vi "Create channel.vi"(8 "error in (no error)":errorcluster, 10 "Lines":T1[](array[typedef])=[1] items=["DIO1...8"=1, "DIO9...16"=2, "DIO17...24"=3, "DIO25...32"=4], 11 "Connection ID":i32=-1) -> (0 "error out":errorcluster, 3 "MicroDAQ.lvlib:Digital output.lvclass":refnum<class "Digital output.lvclass">)   [LabVIEW 2009, in "MicroDAQ.lvlib" / "Digital output.lvclass"]
uses:
  <instrlib>/MicroDAQ/Channel/Digital output/Digital output.lvclass
  <instrlib>/MicroDAQ/Tools/Digital IO channels.ctl
  <instrlib>/MicroDAQ/Channel/Channel.lvclass
  <instrlib>/MicroDAQ/Tools/DIO set direction argument.ctl
  <instrlib>/MicroDAQ/MicroDAQ.lvlib
  <instrlib>/MicroDAQ/Mlink library wraper/mlink.lvlib
  <instrlib>/MicroDAQ/Channel/Digital Input/Digital Input.lvclass
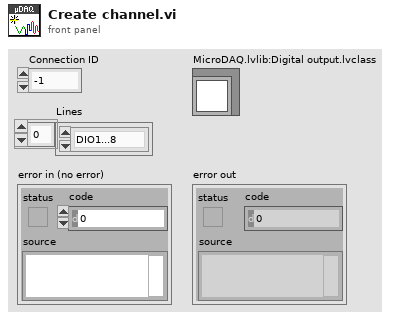
[diagram p1: front panel]
types:
  T1 = typedef "MicroDAQ.lvlib/Digital IO channels.ctl" = u8
  T2 = typedef "MicroDAQ.lvlib/DIO set direction argument.ctl" = enum8{"Input", "Output"}
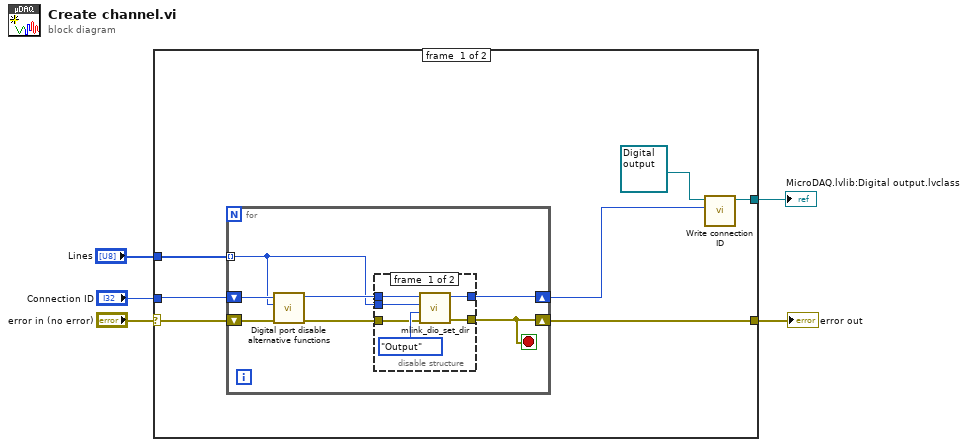
[diagram p0: block diagram]
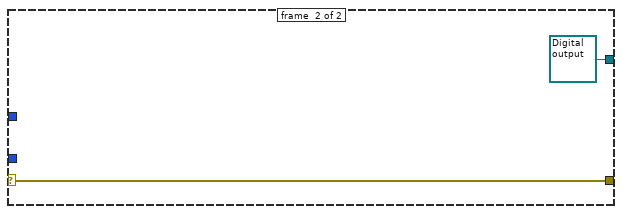
[diagram p3: hidden frame]
diagram:
  n1 = case shown="No Error" "error in (no error)" {
    selector: "error in (no error)" -> [w11 w29]
    tunnel: "Connection ID" -> [w12 _]
    tunnel: "Lines" -> [w10 _]
    tunnel: [w9 w29] -> w3
    tunnel: [w7 refnum<class "Digital output.lvclass"> refnum ("Task out")] -> w1
    frame #0 {
      n2 = for {
        tunnel: w10 -> [w13] mode=indexing
        shift-right: [w16] -> w8
        shift-left: w12 -> [w14]
        shift-right: [w15] -> w9
        shift-left: w11 -> [w19]
        stop <- w15 stop-if-true
        n3 = call <instrlib>:"Digital port disable alternative functions.vi"("error in (no error)"=w19, "Lines"=w13, "Connection ID"=w14) -> ("error out"=w17:errorcluster, "connection ID out"=w18:i32)  [unwired: 7 in]
        n4 = disable-structure shown="Enabled" {
          disable-tunnel: w18 -> [w25 w27]
          disable-tunnel: w17 -> [w23 w26]
          disable-tunnel: [w22 w27] -> w16
          disable-tunnel: [w21 w26] -> w15
          disable-tunnel: w13 -> [w20 _]
          frame #0 {
            n5 = call <instrlib>:"mlink_dio_set_dir.vi"("error in (no error)"=w23, "direction"=DIO_set_direction_argument."Output", "bank"=w20, "connection ID"=w25) -> ("error out"=w21:errorcluster, "connection ID out"=w22:i32)  [unwired: 6 in]
          }
          frame #1 {
          }
        }
      }
      n6 = call <instrlib>:"Write connection ID.vi"("connection ID"=w8, "Task in"=refnum<class "Digital output.lvclass"> refnum ("MicroDAQ.lvlib:Digital output.lvclass")) -> ("Task out"=w7:refnum<class "Digital output.lvclass">)  [unwired: 9 in]
    }
    frame #1 {
    }
  }
  "error out" <- w3
  "MicroDAQ.lvlib:Digital output.lvclass" <- w1
